vi "Begin.vi"(8 "error in":errorcluster) -> (0 "error out":errorcluster)   [LabVIEW 2020]
doc: "Called before other user functions, this VI is expected to open initial I/O refnums, load in file data, and do all program initialization. Notice that the <B>error out</B> terminal is simply used for data flow. Wiring it to other structures or subVIs ensures that this VI runs first."
uses:
  <vilib>/Rock Robotics/WPI/DriverStation/WPI_DriverStationRobotMode2.ctl
  <vilib>/Rock Robotics/WPI/Joystick/WPI_JoystickDeviceEnum.ctl
  <vilib>/Rock Robotics/SystemInterfaces/DIO/FPGA_DIOChannel.ctl
  <vilib>/Rock Robotics/SystemInterfaces/DIO/FPGA_DIORelayChannel.ctl
  <vilib>/Rock Robotics/WPI/Relay/WPI_RelayDirection.ctl
  Robot Global Data.vi
  <vilib>/Rock Robotics/Network Tables/NT Write String Array.vi
  <vilib>/Rock Robotics/WPI/Switch/WPI_SwitchOpenLimit.vi
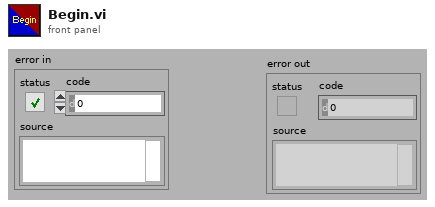
[diagram p1: front panel]
types:
  T1 = typedef "WPI_RelayDirection.ctl" = enum16{"Both directions", "Forward only", "Reverse only"}
  T2 = typedef "FPGA_DIORelayChannel.ctl" = enum8{"Relay 0", "Relay 1", "Relay 2", "Relay 3", "Invalid"}
  T3 = typedef "FPGA_DIOChannel.ctl" = enum8{"DIO 0", "DIO 1", "DIO 2", "DIO 3", "DIO 4", "DIO 5", "DIO 6", "DIO 7", "DIO 8", "DIO 9", "DIO MXP 0", "DIO MXP 1", "DIO MXP 2", "DIO MXP 3", "DIO MXP 4", "DIO MXP 5", "DIO MXP 6", "DIO MXP 7", "DIO MXP 8", "DIO MXP 9", "DIO MXP 10", "DIO MXP 11", "DIO MXP 12", "DIO MXP 13", "DIO MXP 14", "DIO MXP 15", "SPI Port CS1", "SPI Port CS2", "SPI Port CS3", "SPI Port MISO", "SPI Port MOSI", "Invalid"}
  T4 = typedef "WPI_JoystickDeviceEnum.ctl" = enum16{"USB 0", "USB 1", "USB 2", "USB 3", "USB 4", "USB 5"}
  T5 = typedef "WPI_DriverStationRobotMode2.ctl" = enum16{"Autonomous Disabled", "Autonomous Enabled", "Teleop Disabled", "Teleop Enabled", "Disconnected", "Finish", "Test Disabled", "Test Enabled", "Emergency Stopped"}
  T6 = typedef "WPI_JoystickDevRef.ctl" = cluster{"Device":T4}
  T7 = typedef "WPI_SwitchDevRef.ctl" = cluster{"DevStatus":errorcluster, "DIO Channel":T3, "CntIndex":T8, "Normally Closed":bool}
  T8 = typedef "FPGA_CounterCtrSystemIndex.ctl" = enum8{"Ctr 0", "Ctr 1", "Ctr 2", "Ctr 3", "Ctr 4", "Ctr 5", "Ctr 6", "Ctr 7", "Invalid"}
  T9 = typedef "WPI_RelayDevRef.ctl" = cluster{"DevStatus":errorcluster, "Relay Channel":T2, "Relay Direction":T1}
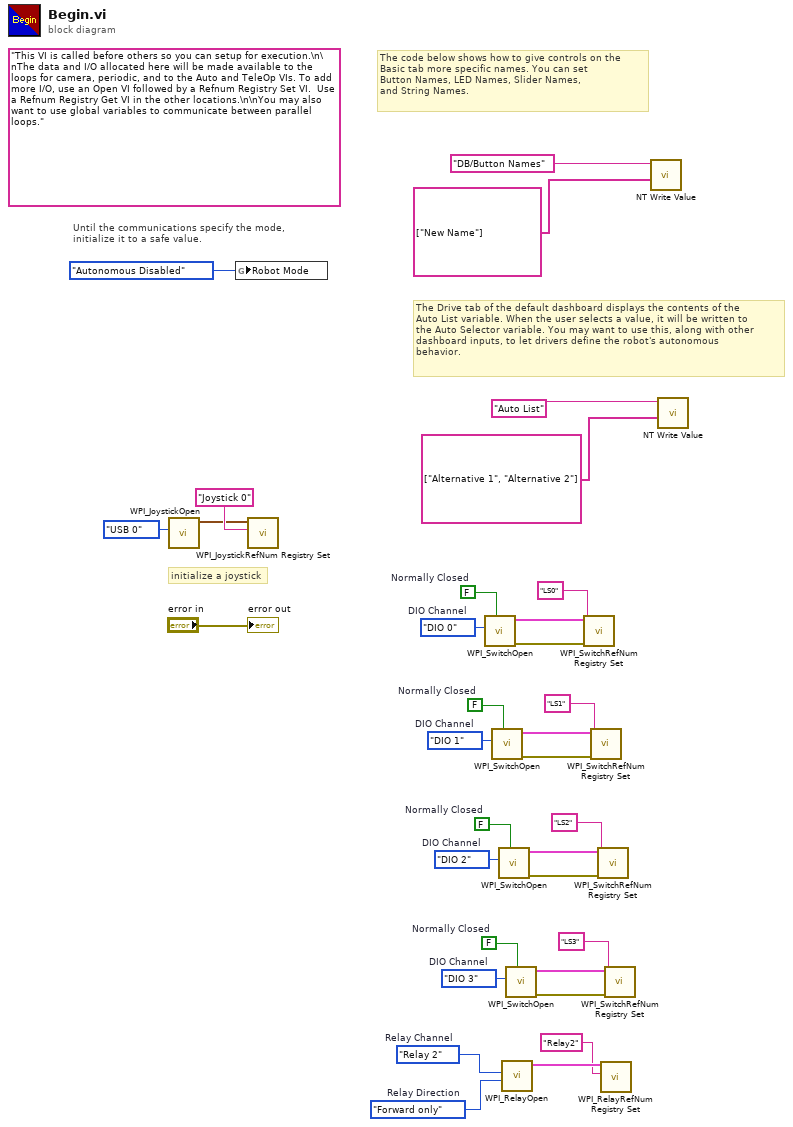
[diagram p0: block diagram]
diagram:
  w1 = WPI_RelayDirection."Forward only"  # Relay Direction
  w2 = FPGA_DIORelayChannel."Relay 2"  # Relay Channel
  w8 = FALSE  # Normally Closed
  w9 = FPGA_DIOChannel."DIO 3"  # DIO Channel
  w13 = FALSE  # Normally Closed
  w14 = FPGA_DIOChannel."DIO 2"  # DIO Channel
  w18 = FALSE  # Normally Closed
  w19 = FPGA_DIOChannel."DIO 1"  # DIO Channel
  w23 = FALSE  # Normally Closed
  w24 = FPGA_DIOChannel."DIO 0"  # DIO Channel
  (unwired) "This VI is called before others so you can setup for execution.\n\nThe data and I/O allocated here will be made available to the loops for camera, periodic, and to the Auto and TeleOp VIs. To add more I/O, use an Open VI followed by a Refnum Registry Set VI.  Use a Refnum Registry Get VI in the other locations.\n\nYou may also want to use global variables to communicate between parallel loops."
  # "The Drive tab of the default dashboard displays the contents of the\nAuto List variable. When the user selects a value, it will be written to\nthe Auto Selector variable. You may want to use this, along with other\ndashboard inputs, to let drivers define the robot's autonomous\nbehavior."
  # "The code below shows how to give controls on the\nBasic tab more specific names. You can set\nButton Names, LED Names, Slider Names,\nand String Names."
  # "initialize a joystick"
  # "Until the communications specify the mode,\ninitialize it to a safe value."
  n1 = call <vilib>:"WPI_JoystickOpen.vi"("JoystickDevice"=WPI_JoystickDeviceEnum."USB 0") -> ("JoystickDevRef"=w31:T6)  [unwired: 10 in]
  n2 = global write "Robot Global Data.vi" "Robot Mode"(WPI_DriverStationRobotMode2."Autonomous Disabled" ("Robot Mode")) -> ()
  n3 = call <vilib>:"WPI_JoystickRefNum Registry Set.vi"("refnum name"="Joystick 0", "JoystickDevRef"=w31) -> ()  [unwired: 8 in, 2 out]
  n4 = call-poly <vilib>:"WPI_SwitchOpen.vi"("Normally Closed"=w23, "DIO Channel"=w24) -> ("error out"=w21:errorcluster, "SwitchDevRef"=w22:T7)  [unwired: 8 in]
  n5 = call-poly <vilib>:"WPI_SwitchOpen.vi"("Normally Closed"=w18, "DIO Channel"=w19) -> ("error out"=w16:errorcluster, "SwitchDevRef"=w17:T7)  [unwired: 8 in]
  n6 = call-poly <vilib>:"WPI_SwitchOpen.vi"("Normally Closed"=w13, "DIO Channel"=w14) -> ("error out"=w11:errorcluster, "SwitchDevRef"=w12:T7)  [unwired: 8 in]
  n7 = call <vilib>:"WPI_RelayOpen.vi"("Relay Direction"=w1, "Relay Channel"=w2) -> ("RelayDevRef"=w4:T9)  [unwired: 8 in, 1 out]
  n8 = call-poly <vilib>:"WPI_SwitchOpen.vi"("Normally Closed"=w8, "DIO Channel"=w9) -> ("error out"=w6:errorcluster, "SwitchDevRef"=w7:T7)  [unwired: 8 in]
  n9 = call <vilib>:"WPI_SwitchRefNum Registry Set.vi"("error in (no error)"=w21, "refnum name"="LS0", "SwitchDevRef"=w22) -> ()  [unwired: 7 in, 2 out]
  n10 = call <vilib>:"WPI_SwitchRefNum Registry Set.vi"("error in (no error)"=w16, "refnum name"="LS1", "SwitchDevRef"=w17) -> ()  [unwired: 7 in, 2 out]
  n11 = call <vilib>:"WPI_SwitchRefNum Registry Set.vi"("error in (no error)"=w11, "refnum name"="LS2", "SwitchDevRef"=w12) -> ()  [unwired: 7 in, 2 out]
  n12 = call <vilib>:"WPI_RelayRefNum Registry Set.vi"("refnum name"="Relay2", "RelayDevRef"=w4) -> ()  [unwired: 8 in, 2 out]
  n13 = call <vilib>:"WPI_SwitchRefNum Registry Set.vi"("error in (no error)"=w6, "refnum name"="LS3", "SwitchDevRef"=w7) -> ()  [unwired: 7 in, 2 out]
  n14 = call-poly <vilib>:"NT Write Value.vi"("value"=string[] ["New Name"], "name"="DB/Button Names" ("Name")) -> ()  [unwired: 9 in, 1 out]
  n15 = call-poly <vilib>:"NT Write Value.vi"("value"=string[] ["Alternative 1", "Alternative 2"] ("String Array"), "name"="Auto List" ("Name")) -> ()  [unwired: 9 in, 1 out]
  "error out" <- "error in"
